vi "Drawing Not New Line.vi"() -> ()   [LabVIEW 2021]
uses:
  <vilib>/Utility/inputDevices.llb/closeMouse.vi
  <vilib>/Utility/inputDevices.llb/mouseAcquire.vi
panel:
  out "XY Graph":cluster{"Y":dbl[], "Y":dbl[]}[](graph)
  out "button info":T1
  in  "stop":bool
  out "axis info":T2
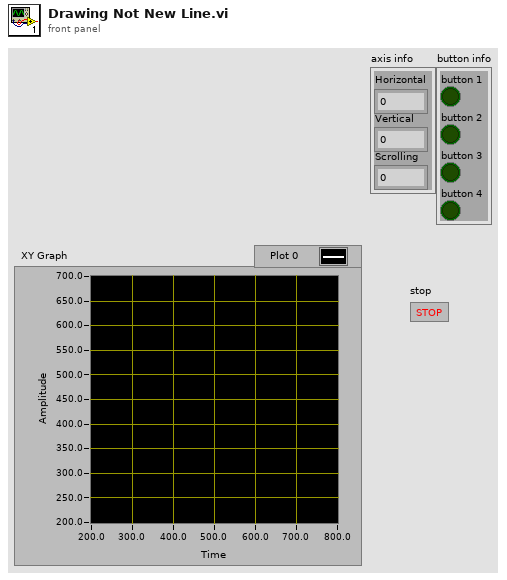
[diagram p1: front panel]
types:
  T1 = cluster{"button 1":bool, "button 2":bool, "button 3":bool, "button 4":bool}
  T2 = cluster{"Horizontal":i32, "Vertical":i32, "Scrolling":i32}
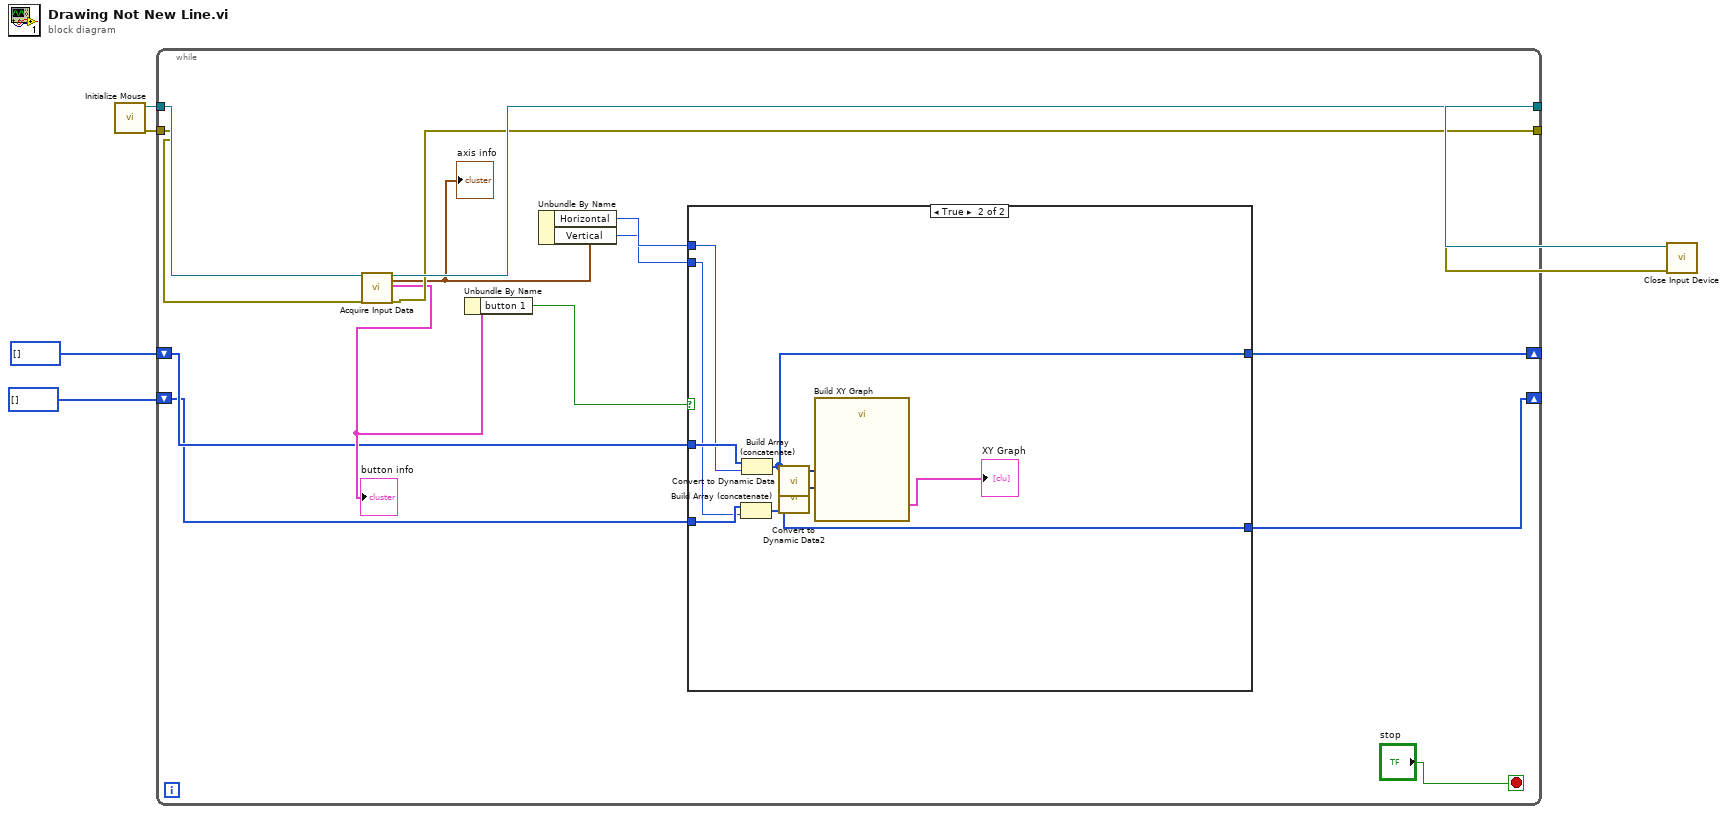
[diagram p0: block diagram]
diagram:
  n1 = call <vilib>:"Initialize Mouse.vi"() -> ("error out"=w5:errorcluster, "device ID"=w6:refnum<k1>)  [unwired: 10 in]
  n2 = while {
    tunnel: w6 -> [w19]
    tunnel: w5 -> [w18]
    tunnel: [w17] -> w4
    tunnel: [w16] -> w3
    shift-right: [w7] -> _
    shift-left: i32[] [] -> [w10]
    shift-right: [w8] -> _
    shift-left: i32[] [] -> [w9]
    stop <- "stop" stop-if-true
    n3 = call-poly <vilib>:"Acquire Input Data.vi"("device ID"=w19, "error in (no error)"=w18) -> ("device ID"=w17:refnum<k1>, "axis info"=w13:T2, "button info"=w15:T1, "error out"=w16:errorcluster)  [unwired: 14 in]
    "button info" <- w15
    "axis info" <- w13
    n4 = Unbundle By Name(w15) -> ("button 1"=w14:bool)
    n5 = Unbundle By Name(w13) -> ("Horizontal"=w12:i32, "Vertical"=w11:i32)
    n6 = case shown="True" w14 {
      tunnel: w12 -> [_ w29]
      tunnel: w11 -> [_ w27]
      tunnel: w10 -> [w22 w30]
      tunnel: w9 -> [w21 w28]
      tunnel: [w21 w24] -> w8
      tunnel: [w22 w23] -> w7
      frame False {
      }
      frame True {
        n7 = Build Array (concatenate)(w28, w27) -> (w24:i32[])
        n8 = Build Array (concatenate)(w30, w29) -> (w23:i32[])
        n9 = call "Convert to Dynamic Data"("Array"=w23) -> ("Dynamic Data Type"=w26:dynamicdata)  [unwired: 3 in]
        n10 = call "Convert to Dynamic Data2"("Array"=w24) -> ("Dynamic Data Type"=w25:dynamicdata)  [unwired: 3 in]
        n11 = call "Build XY Graph"("Y Input"=w25, "X Input"=w26) -> ("XY Graph"=→"XY Graph":cluster{"X":dbl[], "Y":dbl[]}[])  [unwired: 8 in, 1 out]
      }
    }
  }
  n12 = call-poly <vilib>:"Close Input Device.vi"("error in (no error)"=w3, "device ID"=w4) -> ()  [unwired: 8 in, 1 out]
